vi "CC create observation queue.vi"(8 "error in (no error)":errorcluster) -> (0 "error out":errorcluster, 3 "Observation Queue":refnum<queue>)   [LabVIEW 2021]
uses:
  Subsystems/SS cluster Script Status Queue.ctl
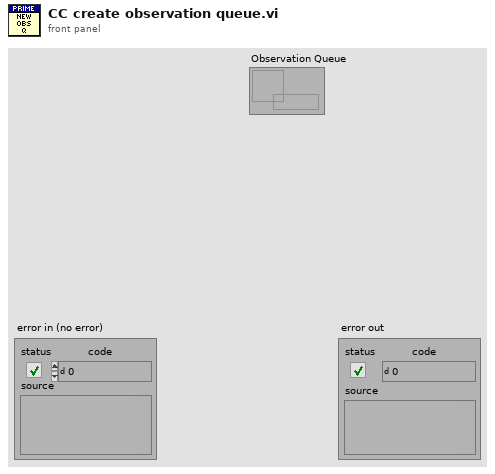
[diagram p1: front panel]
types:
  T1 = typedef "SS cluster Script Status Queue.ctl" = cluster{"Msg":string, "Data":variant}
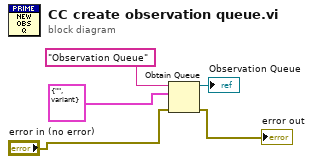
[diagram p0: block diagram]
diagram:
  n1 = Obtain Queue(name (unnamed)="Observation Queue", element data type=T1 {"Msg"="", "Data"=variant} ("Data Q"), error in (no error)="error in (no error)") -> (queue out=→"Observation Queue":refnum<queue>, error out=→"error out":errorcluster)  [unwired: 2 in, 1 out]
